vi "HFR500 Get Live FIDs.vi"() -> (1 "Available Channels":string[](array[string]))   [LabVIEW 2022 SP3]
uses:
  Globals/Meas_global.vi
panel:
  out "Array 2":string[](array[string])
  out "Channel above 200deg":string[](array[string])
  out "Array":string[](array[string])
  out "filenames":string[](array[string])
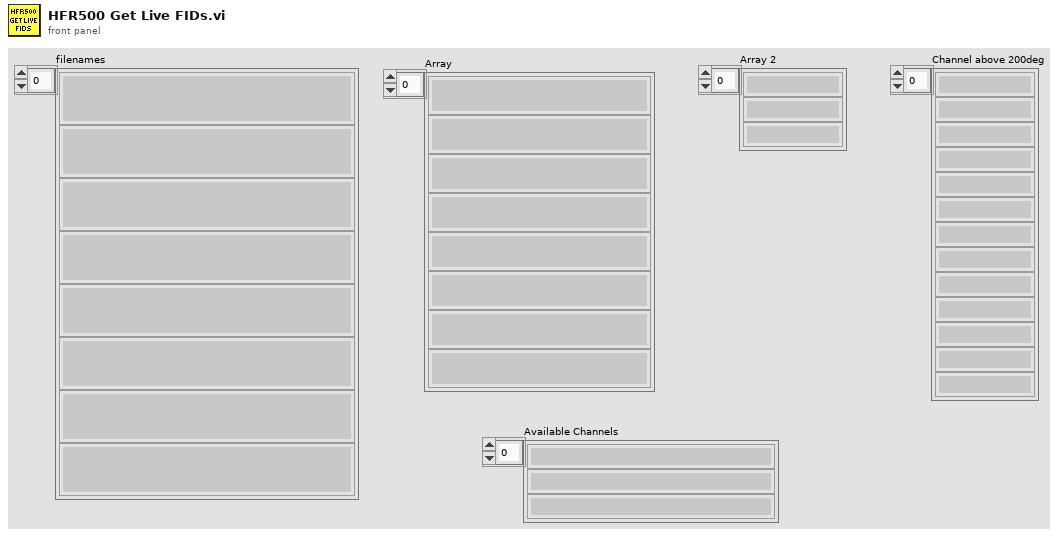
[diagram p1: front panel]
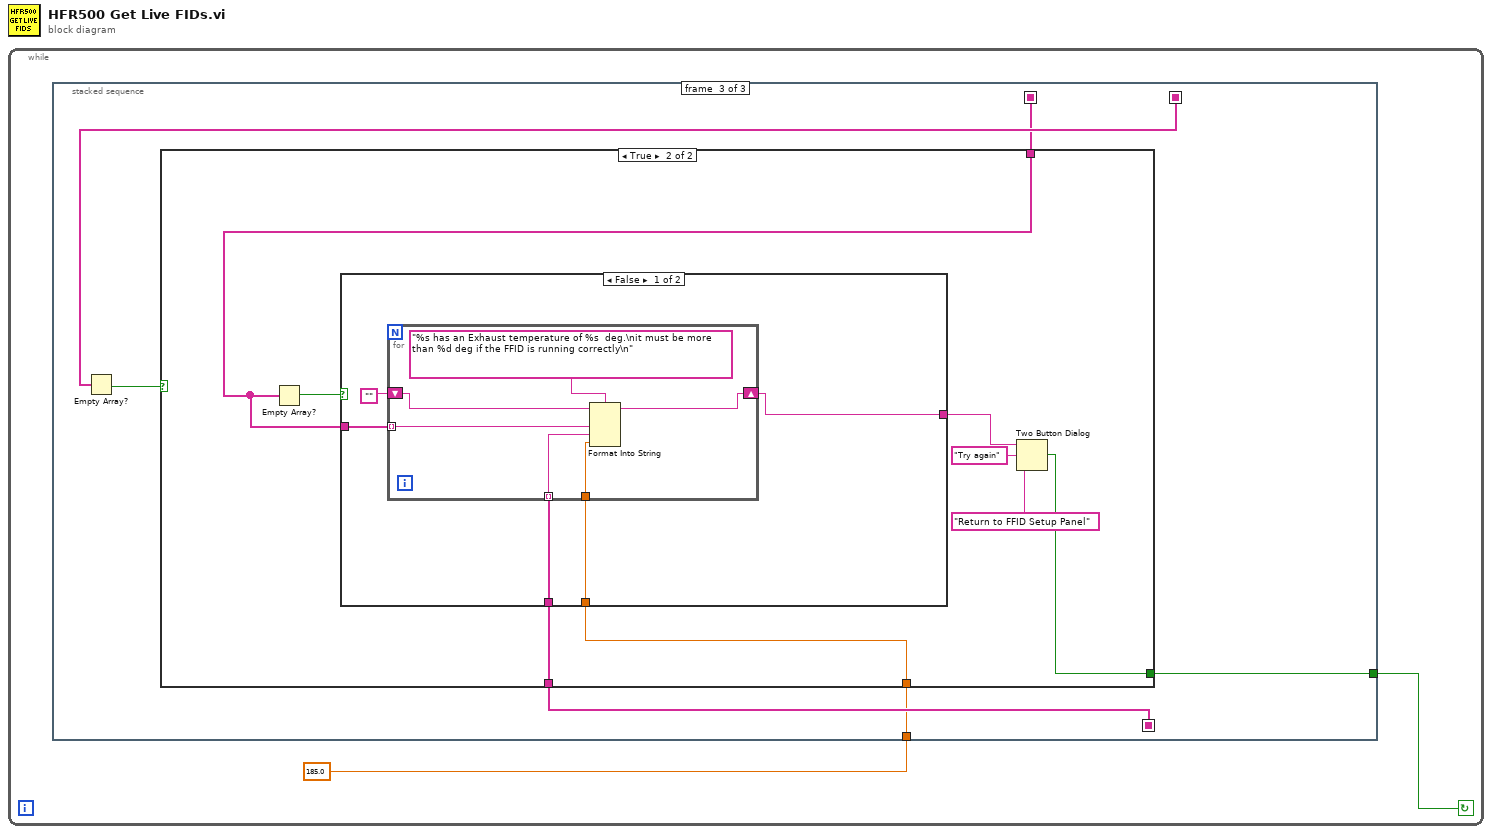
[diagram p0: block diagram]
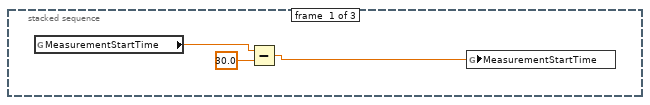
[diagram p2: hidden frame]
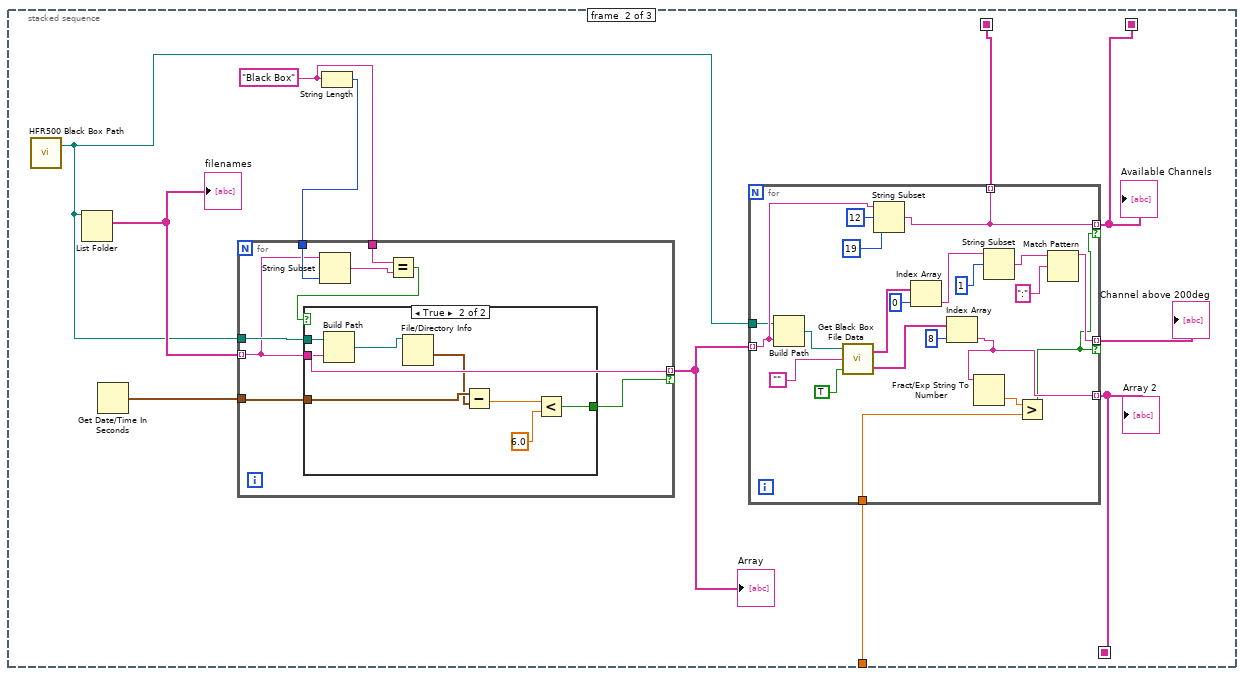
[diagram p3: hidden frame]
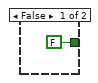
[diagram p4: hidden frame]
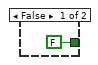
[diagram p5: hidden frame]
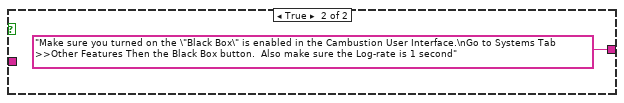
[diagram p6: hidden frame]
diagram:
  n1 = while {
    stop <- w2 continue-if-true
    n2 = stacked-sequence {
      seq-local: [_ w9 _] -> [_ _ w60]
      seq-local: [_ w8 _] -> [_ _ w58]
      seq-local: [_ w7 _] -> [_ _ w57]
      tunnel: [_ _ w56] -> w2
      tunnel: 185.0 ("y") -> [_ w6 w55]
      frame #0 {
        n3 = global read "Meas_global.vi" "MeasurementStartTime"() -> (w5:dbl)
        n4 = Subtract(x=w5, y=30.0) -> (x-y=w3:dbl)
        n5 = global write "Meas_global.vi" "MeasurementStartTime"(w3) -> ()
      }
      frame #1 {
        w13 = "Black Box"
        n6 = call "HFR500 Black Box Path.vi"() -> ("Black Box Folder"=w11:path)  [unwired: 2 in, 1 out]
        n7 = List Folder(path=w11) -> (filenames=w16:string[])  [unwired: 3 in, 3 out]
        "filenames" <- w16
        n8 = Get Date/Time In Seconds() -> (seconds since 1Jan1904=w15:timestamp)
        n9 = String Length(string=w13) -> (length=w14:i32)
        n10 = for {
          tunnel: w11 -> [w45]
          tunnel: w16 -> [w41] mode=indexing
          tunnel: w15 -> [w44]
          tunnel: [w41] -> w12 mode=indexing if=w43
          tunnel: w14 -> [w42]
          tunnel: w13 -> [w39]
          n11 = String Subset(string=w41, length (rest)=w42) -> (substring=w40:string)  [unwired: 1 in]
          n12 = Equal?(x=w39, y=w40) -> (x = y?=w38:bool)
          n13 = case shown="True" w38 {
            tunnel: w45 -> [_ w54]
            tunnel: w44 -> [_ w48]
            tunnel: [FALSE w50] -> w43
            tunnel: w41 -> [_ w49]
            frame False {
            }
            frame True {
              n14 = Build Path(base path=w54, name or relative path=w49) -> (appended path=w53:path)
              n15 = File/Directory Info(path=w53) -> (last mod=w47:timestamp)  [unwired: 1 in, 6 out]
              n16 = Subtract(x=w48, y=w47) -> (x-y=w52:dbl)
              n17 = Less?(x=w52, y=6.0) -> (x < y?=w50:bool)
            }
          }
        }
        "Array" <- w12
        n18 = for {
          tunnel: w12 -> [w22] mode=indexing
          tunnel: w11 -> [w20]
          tunnel: [w26] -> w10 mode=indexing if=w21
          tunnel: [w25] -> w7 mode=indexing
          tunnel: [w18] -> w9 mode=indexing if=w21
          tunnel: [w18] -> w8 mode=indexing
          tunnel: w6 -> [w17]
          n19 = Build Path(base path=w20, name or relative path=w22) -> (appended path=w19:path)
          n20 = call "Get Black Box File Data.vi"("Delete File?"=TRUE, "Inst Name"="", "Black Box Filename"=w19) -> ("Channel Values"=w35:string[], "Channel Names"=w32:string[])
          n21 = String Subset(string=w22, offset (0)=12, length (rest)=19 ("length (rest)")) -> (substring=w18:string)
          n22 = Index Array(array=w32, index=0) -> (element=w30:string)
          n23 = Index Array(array=w35, index=8) -> (element=w25:string)
          n24 = Fract/Exp String To Number(string=w25) -> (number=w34:dbl)  [unwired: 3 in, 1 out]
          n25 = String Subset(string=w30, offset (0)=1) -> (substring=w28:string)  [unwired: 1 in]
          n26 = Greater?(x=w34, y=w17) -> (0:w21:bool)
          n27 = Match Pattern(string=w28, regular expression=":") -> (before substring=w26:string)  [unwired: 1 in, 3 out]
        }
        "Channel above 200deg" <- w10
        "Array 2" <- w7
        "Available Channels" <- w9
      }
      frame #2 {
        n28 = Empty Array?(array=w60) -> (empty?=w59:bool)
        n29 = case shown="True" w59 {
          tunnel: w58 -> [_ w67]
          tunnel: w57 -> [_ w66]
          tunnel: [FALSE ("T button?") w65] -> w56
          tunnel: w55 -> [_ w62]
          frame False {
          }
          frame True {
            n30 = Empty Array?(array=w67) -> (empty?=w69:bool)
            n31 = case shown="False" w69 {
              tunnel: [w71 "Make sure you turned on the \"Black Box\" is enabled in the Cambustion User Interface.\nGo to Systems Tab >>Other Features Then the Black Box button.  Also make sure the Log-rate is 1 second"] -> w68
              tunnel: w67 -> [w74 _]
              tunnel: w66 -> [w73 _]
              tunnel: w62 -> [w70 _]
              frame False {
                n32 = for {
                  tunnel: w74 -> [w80] mode=indexing
                  tunnel: w73 -> [w79] mode=indexing
                  shift-right: [w77] -> w71
                  shift-left: "" -> [w76]
                  tunnel: w70 -> [w75]
                  n33 = Format Into String(format string="%s has an Exhaust temperature of %s  deg.\nit must be more than %d deg if the FFID is running correctly\n", initial string=w76, w80, w79, w75) -> (resulting string=w77:string)  [unwired: 1 in, 1 out]
                }
              }
              frame True {
              }
            }
            n34 = Two Button Dialog(message=w68, 1:"Return to FFID Setup Panel" ("F button name (\"Cancel\")"), 2:"Try again" ("T button name (\"OK\")")) -> (T button?=w65:bool)
          }
        }
      }
    }
  }
